vi "Line Creator Indicator.vi"(10 "x":i32, 11 "Image":T1) -> (3 "Image Out":T1)   [LabVIEW 2013]
uses:
  <vilib>/vision/Image Controls.llb/IMAQ Image.ctl
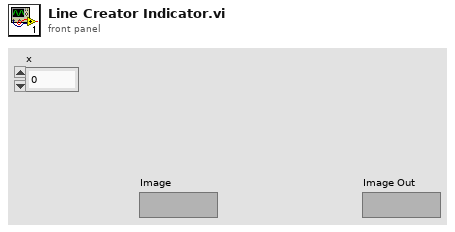
[diagram p1: front panel]
types:
  T1 = typedef "IMAQ Image.ctl" = refnum<image>
  T2 = cluster{cluster{i32, i32}, cluster{"X Resolution":i32, i32}}
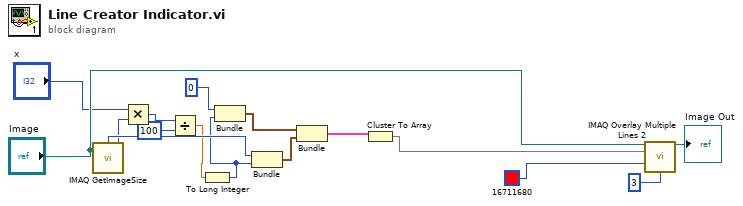
[diagram p0: block diagram]
diagram:
  n1 = call "IMAQ GetImageSize"("Image"="Image") -> ("Y Resolution"=w9:i32, "X Resolution"=w10:i32)  [unwired: 3 in, 1 out]
  n2 = Multiply(x="x", y=w9) -> (x*y=w8:i32)
  n3 = Divide(x=w8, y=100) -> (x/y=w6:dbl)
  n4 = To Long Integer(number=w6) -> (32bit integer=w5:i32)
  n5 = Bundle(0, w5) -> (w16:cluster{i32, i32})  [unwired: 1 in]
  n6 = Bundle("X Resolution"=w10, w5) -> (w15:cluster{"X Resolution":i32, i32})  [unwired: 1 in]
  n7 = Bundle(w16, w15) -> (w14:T2)  [unwired: 1 in]
  n8 = Cluster To Array(cluster=w14) -> (array=w13:cluster{"X Resolution":i32, i32}[])
  n9 = call "IMAQ Overlay Multiple Lines 2"("Image"="Image", "Line End Points"=w13, "Color"=u32 16711680, "Width"=u32 3) -> ("Image Out"=→"Image Out":T1)  [unwired: 10 in, 1 out]
